vi "Property Tree.vi"() -> ()   [LabVIEW 2019]
doc: "This example shows how to refresh modules and read different properties of EtherCAT masters and devices. A tree control is used to display all EtherCAT masters and devices, as well as their properties. EtherCAT masters are sorted by master ids. Devices are sorted by position addresses."
uses:
  <resource>/objmgr/IndComECAT.rc
  <resource>/objmgr/cRIO.rc
panel:
  in  "properties of refreshed master and slave":string(tree)
  # "Overview: Demonstrates how to refresh modules and read different properties of EtherCAT masters and devices.\nRequirements: NI-Industrial Communications for EtherCAT, LabVIEW Real-Time Module, NI-RIO Device Drivers. \nInstructions:\n1. Right-click RT Target in the project explorer and select Properties from the shortcut menu. In the Real-Time CompactRIO Properties dialog box that appears, click the General tab and specify the IP address of the RT Target that you use.\n2. Run this VI."
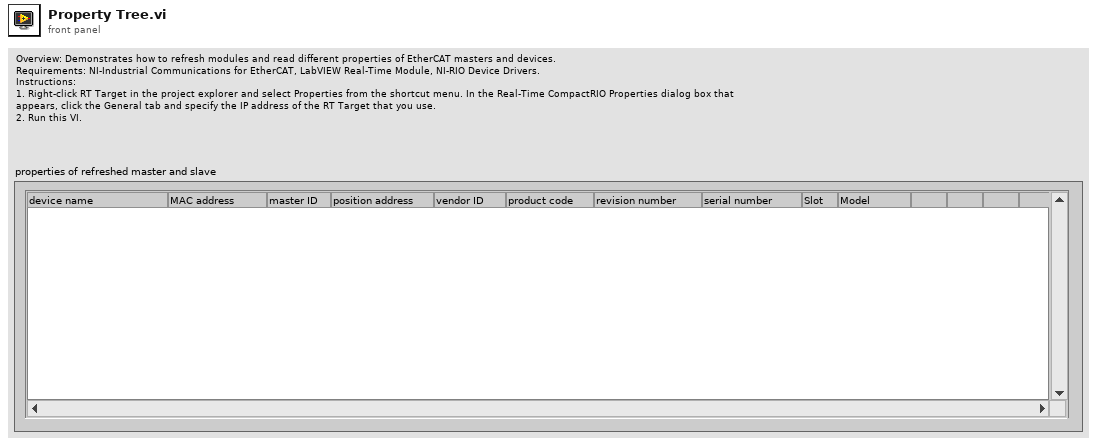
[diagram p1: front panel]
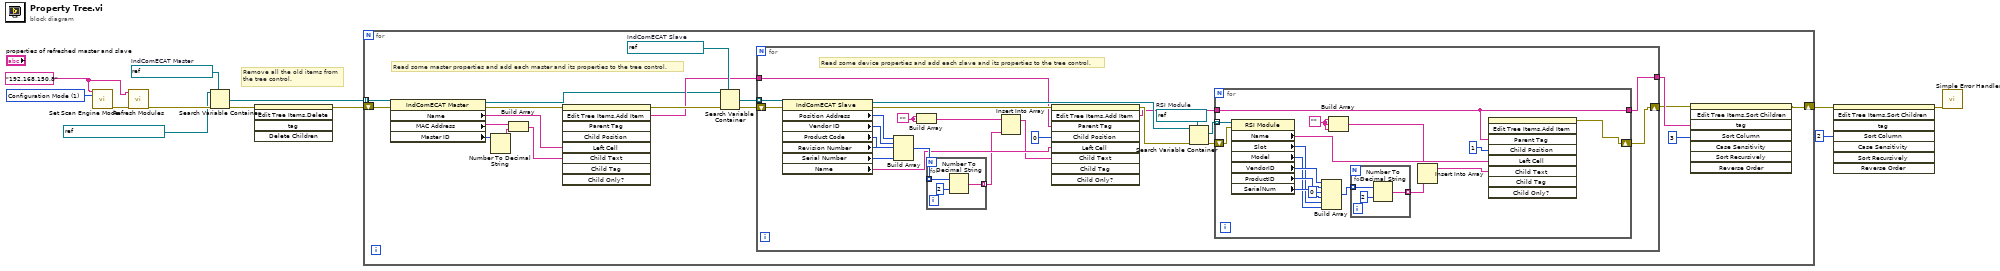
[diagram p0: block diagram]
diagram:
  w2 = "192.168.150.8" ("target address (localhost)")
  w7 = 1 items=["Configuration Mode"=1, "Active Mode"=2] ("mode (Active Mode)")
  w5 = refnum<k21> refnum  # IndComECAT Master
  # "Remove all the old items from\nthe tree control."
  n1 = call <vilib>:"Set Scan Engine Mode.vi"("target address (localhost)"=w2, "mode (Active Mode)"=w7) -> ("error out"=w6:errorcluster)  [unwired: 13 in]
  n2 = call <vilib>:"Refresh Modules.vi"("error in (no error)"=w6, "target address (localhost)"=w2) -> ("error out"=w8:errorcluster)  [unwired: 9 in]
  n3 = Search Variable Container(7:w5, 8:w8, 11:refnum<k21> "ni.var.psp://192.168.150.8" ("container refnum in")) -> (0:w9:errorcluster, 2:w11:refnum<k21>[])  [unwired: 3 in, 1 out]
  n4 = invoke on="properties of refreshed master and slave" class="Tree (strict)" method="Edit Tree Items.Delete"(error in=w9) -> (error out=w10:errorcluster)  [unwired: 4 in, 4 out]
  n5 = for {
    tunnel: w11 -> [w27] mode=indexing
    shift-right: [w16] -> w3
    shift-left: w10 -> [w29]
    w26 = refnum<k21> refnum  # IndComECAT Slave
    # "Read some master properties and add each master and its properties to the tree control."
    n6 = property class="IndComECAT Master"(reference=w27, error in=w29) -> (reference out=w14:refnum<k21>, error out=w28:errorcluster, "Name"=w19:string, "MAC Address"=w20:string, "Master ID"=w21:u32)
    n7 = Number To Decimal String(number=w21) -> (decimal integer string=w30:string)  [unwired: 1 in]
    n8 = Build Array(w20, w30) -> (w18:string[])
    n9 = invoke on="properties of refreshed master and slave" class="Tree (strict)" method="Edit Tree Items.Add Item"(error in=w28, "Left Cell"=w19, "Child Text"=w18) -> (error out=w25:errorcluster, "Edit Tree Items:Add Item"=w22:string)  [unwired: 6 in, 7 out]
    n10 = Search Variable Container(7:w26, 8:w25, 11:w14) -> (0:w23:errorcluster, 2:w24:refnum<k21>[])  [unwired: 3 in, 1 out]
    n11 = for {
      tunnel: w24 -> [w54] mode=indexing
      tunnel: w22 -> [w36]
      tunnel: [w34] -> w17
      shift-right: [w32] -> w15
      shift-left: w23 -> [w51]
      w38 = refnum<k21> refnum  # RSI Module
      w49 = "" ("Name")
      # "Read some device properties and add each slave and its properties to the tree control."
      n12 = property class="IndComECAT Slave"(reference=w54, error in=w51) -> (reference out=w39:refnum<k21>, error out=w50:errorcluster, "Position Address"=w41:u16, "Vendor ID"=w42:u32, "Product Code"=w43:u32, "Revision Number"=w44:u32, "Serial Number"=w45:u32, "Name"=w52:string)
      n13 = Build Array(w41, w42, w43, w44, w45) -> (w53:u32[])
      n14 = Build Array(w49, w49) -> (w48:string[])
      n15 = for {
        tunnel: w53 -> [w77] mode=indexing
        tunnel: [w76] -> w47 mode=indexing
        n16 = Number To Decimal String(number=w77, width (-)=i16 2) -> (decimal integer string=w76:string)
      }
      n17 = Insert Into Array(array=w48, new element=w47) -> (w46:string[])  [unwired: 1 in]
      n18 = invoke on="properties of refreshed master and slave" class="Tree (strict)" method="Edit Tree Items.Add Item"(error in=w50, "Parent Tag"=w36, "Child Position"=0, "Left Cell"=w52, "Child Text"=w46) -> (error out=w35:errorcluster, "Edit Tree Items:Add Item"=w31:string)  [unwired: 4 in, 7 out]
      n19 = Search Variable Container(7:w38, 8:w35, 11:w39) -> (0:w33:errorcluster, 2:w37:refnum<k21>[])  [unwired: 3 in, 1 out]
      n20 = for {
        tunnel: w37 -> [w71] mode=indexing
        tunnel: w31 -> [w57]
        tunnel: [w57] -> w34
        shift-right: [w55] -> w32
        shift-left: w33 -> [w56]
        w64 = "" ("Name")
        n21 = property class="RSI Module"(reference=w71, error in=w56) -> ("Name"=w69:string, "Slot"=w58:u32, "Model"=w59:u32, "VendorID"=w63:u32, "ProductID"=w62:u32, "SerialNum"=w61:u32)  [unwired: 2 out]
        n22 = Build Array(w63, w62, u32 0 ("element"), w61, w58, w59) -> (w67:u32[])
        n23 = Build Array(w64, w64, w64) -> (w68:string[])
        n24 = for {
          tunnel: w67 -> [w72] mode=indexing
          tunnel: [w74] -> w66 mode=indexing
          n25 = Number To Decimal String(number=w72, width (-)=i16 2) -> (decimal integer string=w74:string)
        }
        n26 = Insert Into Array(array=w68, new element=w66) -> (w65:string[])  [unwired: 1 in]
        n27 = invoke on="properties of refreshed master and slave" class="Tree (strict)" method="Edit Tree Items.Add Item"("Parent Tag"=w57, "Child Position"=1, "Left Cell"=w69, "Child Text"=w65) -> (error out=w55:errorcluster)  [unwired: 5 in, 8 out]
      }
    }
    n28 = invoke on="properties of refreshed master and slave" class="Tree (strict)" method="Edit Tree Items.Sort Children"(error in=w15, "tag"=w17, "Sort Column"=3) -> (error out=w16:errorcluster)  [unwired: 5 in, 7 out]
  }
  n29 = invoke on="properties of refreshed master and slave" class="Tree (strict)" method="Edit Tree Items.Sort Children"(error in=w3, "Sort Column"=2) -> (error out=w4:errorcluster)  [unwired: 6 in, 7 out]
  n30 = call <vilib>:"Simple Error Handler.vi"("error in (no error)"=w4) -> ()  [unwired: 4 in, 5 out]
